vi "PXI-Set AI Gains by Channel.vi"(0 "AI Channels":u16[](array[numeric]), 5 "Gain":dbl[](array[numeric]), 11 "error in (no error)":errorcluster) -> (15 "error out":errorcluster)   [LabVIEW 2015]
uses:
  PXI Globals.vi
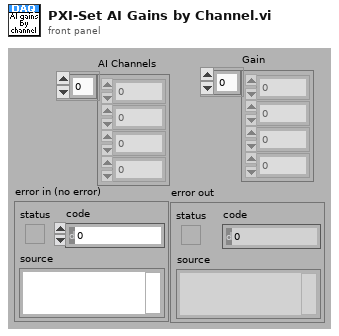
[diagram p1: front panel]
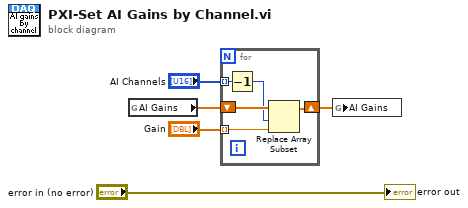
[diagram p0: block diagram]
diagram:
  n1 = global read "PXI Globals.vi" "AI Gains"() -> (w5:dbl[])
  n2 = for {
    shift-right: [w9] -> w4
    shift-left: w5 -> [w10]
    tunnel: "AI Channels" -> [w7] mode=indexing
    tunnel: "Gain" -> [w8] mode=indexing
    n3 = Decrement(x=w7) -> (x-1=w6:u16)
    n4 = Replace Array Subset(array=w10, new element=w8, index=w6) -> (w9:dbl[])
  }
  n5 = global write "PXI Globals.vi" "AI Gains"(w4) -> ()
  "error out" <- "error in (no error)"
